vi "Page_Info_Read.vi"(6 "ctlReferences":T1, 8 "error in (no error)":errorcluster, 11 "Build in":refnum<class "AB_Build.lvclass">) -> (0 "error out":errorcluster, 3 "Build out":refnum<class "AB_Build.lvclass">)   [LabVIEW 2020, in "AB_Deployment.lvlib"]
uses:
  <vilib>/AppBuilder/AB_Classes/Deployment/AB_Deployment.lvlib
  <vilib>/AppBuilder/AB_Classes/Build/AB_Build.lvclass
  <resource>/Framework/Providers/Builds/AppBuilder/AB_UI_Page_Info_References.ctl
  <vilib>/AppBuilder/AB_Classes/Build/AB_Build.lvclass/AB_Build.ctl
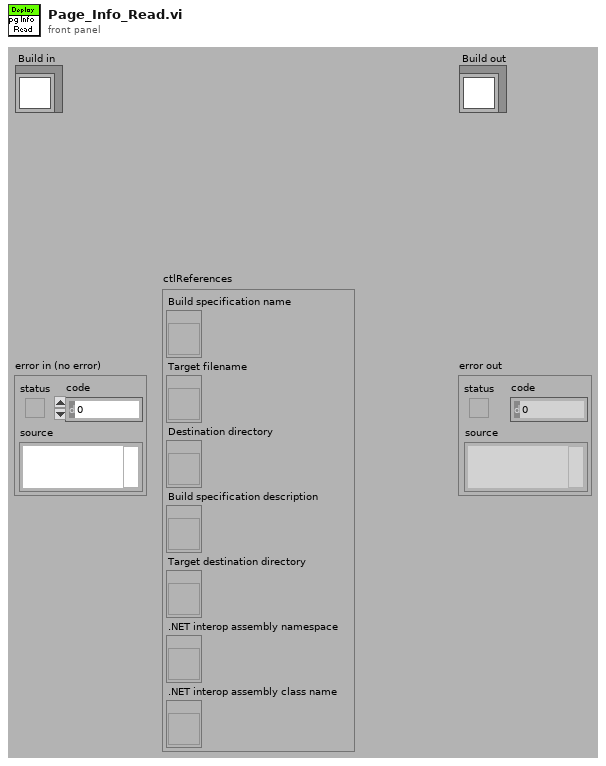
[diagram p1: front panel]
types:
  T1 = typedef "AB_UI_Page_Info_References.ctl" = cluster{"Build specification name":refnum<vi>, "Target filename":refnum<vi>, "Destination directory":refnum<vi>, "Build specification description":refnum<vi>, "Target destination directory":refnum<vi>, ".NET interop assembly namespace":refnum<vi>, ".NET interop assembly class name":refnum<vi>}
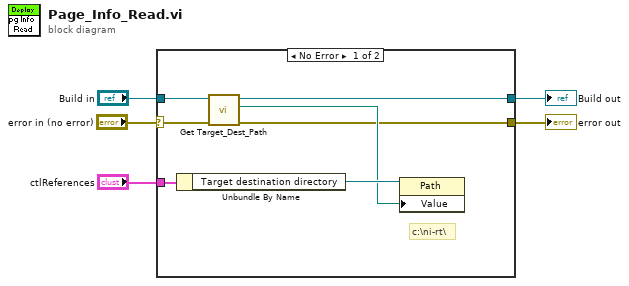
[diagram p0: block diagram]
diagram:
  n1 = case shown="No Error" "error in (no error)" {
    selector: "error in (no error)" -> [w8 w14]
    tunnel: [w9 w14] -> w3
    tunnel: "Build in" -> [w7 w13]
    tunnel: "ctlReferences" -> [w11 _]
    tunnel: [w6 w13] -> w4
    frame No Error {
      # "c:\\ni-rt\\"
      n2 = Unbundle By Name(w11) -> ("Target destination directory"=w12:refnum<vi>)
      n3 = call <vilib>:"Get Target_Dest_Path.vi"("error in (no error)"=w8, "AB_Build in"=w7) -> ("error out"=w9:errorcluster, "Target Dest Path"=w10:path, "AB_Build out"=w6:refnum<class "AB_Build.lvclass">)  [unwired: 7 in]
      n4 = property class="Path"(reference=w12, "Value"=w10) -> ()  [unwired: 1 in, 2 out]
    }
    frame Error {
    }
  }
  "error out" <- w3
  "Build out" <- w4
